vi "Read SA Pin.vi"(8 "error in (no error)":errorcluster, 11 "SpecAn_IM3 in":refnum<class "SpecAn_IM3.lvclass">) -> (0 "error out":errorcluster, 2 "SA Pin":string, 3 "SpecAn_IM3 out":refnum<class "SpecAn_IM3.lvclass">)   [LabVIEW 2018, in "SeqAuto Evaluations.lvlib" / "SpecAn_IM3.lvclass"]
uses:
  SpecAn_IM3.lvclass
  SpecAn_IM3.lvclass/SpecAn_IM3.ctl
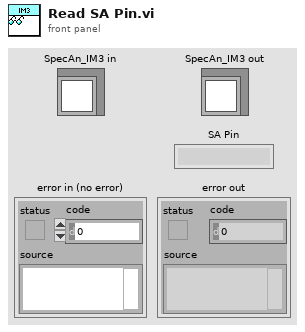
[diagram p1: front panel]
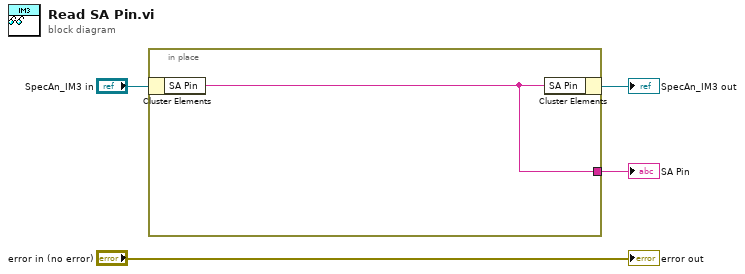
[diagram p0: block diagram]
diagram:
  n1 = in-place {
    in-place-border: [w5] -> w1
    n2 = in-place-cluster #1("SpecAn_IM3 in") -> ("SA Pin"=w5:string)
    n3 = in-place-cluster #1("SA Pin"=w5) -> (→"SpecAn_IM3 out":refnum<class "SpecAn_IM3.lvclass">)
  }
  "SA Pin" <- w1
  "error out" <- "error in (no error)"
